vi "Calibration to List.vi"(8 "error in (no error)":errorcluster, 11 "Calibration":refnum<vi>[](array[refnum])) -> (0 "error out":errorcluster, 3 "List":string)   [LabVIEW 2019, in "Inst.TC.lvclass"]
uses:
  Inst.TC.lvclass
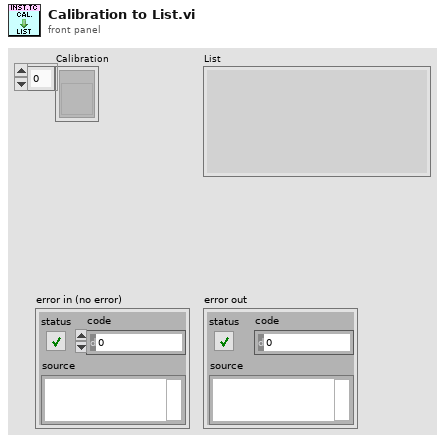
[diagram p1: front panel]
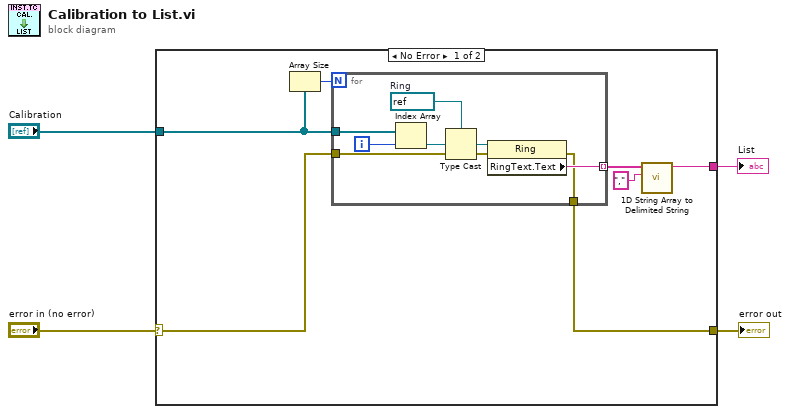
[diagram p0: block diagram]
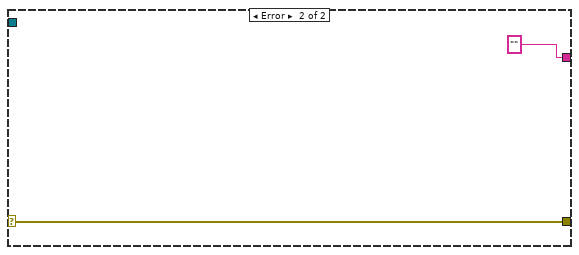
[diagram p2: hidden frame]
diagram:
  n1 = case shown="No Error" "error in (no error)" {
    selector: "error in (no error)" -> [w5 w21]
    tunnel: [w11 "" ("delimited string")] -> w4
    tunnel: [w7 w21] -> w3
    tunnel: "Calibration" -> [w6 _]
    frame No Error {
      n2 = Array Size(array=w6) -> (size(s)=w8:i32)
      n3 = for {
        N: w8 -> [_]
        tunnel: w6 -> [w15]
        tunnel: [w17] -> w9 mode=indexing
        tunnel: w5 -> [w14]
        tunnel: [w13] -> w7
        i -> [w12]
        w19 = refnum<vi> refnum  # Ring
        n4 = Index Array(array=w15, index=w12) -> (element=w16:refnum<vi>)
        n5 = Type Cast(type=w19, x=w16) -> (*(type *) &x=w18:refnum<vi>)
        n6 = property class="Ring"(reference=w18, error in=w14) -> (error out=w13:errorcluster, "RingText.Text"=w17:string)  [unwired: 1 out]
      }
      n7 = call <vilib>:"1D String Array to Delimited String.vi"("delimiter"=",", "string array"=w9) -> ("delimited string"=w11:string)  [unwired: 9 in]
    }
    frame Error {
    }
  }
  "List" <- w4
  "error out" <- w3
